vi "en.vi"   [LabVIEW 2020]
uses:
  88c864df-a670-4eb2-958f-2a5a04899984.vi
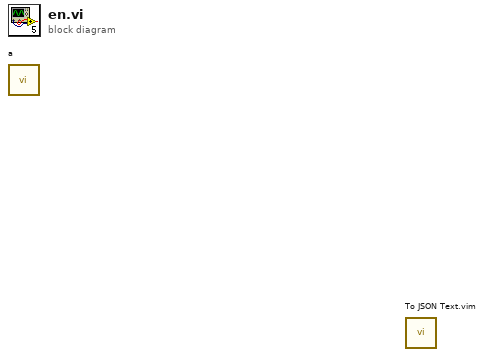
[diagram p0: block diagram]
diagram:
  n1 = call "a.vi"() -> ()  [unwired: 12 in]
  n2 = call "To JSON Text.vim"() -> ()  [unwired: 10 in, 2 out]
